vi "Signal Generator.vi"(0 "Cluster":cluster{"Frequency":dbl, "Amplitude":dbl}) -> ()   [LabVIEW 2015]
panel:
  out "error in":errorcluster
  out "error out":errorcluster
  in  "Stop":bool
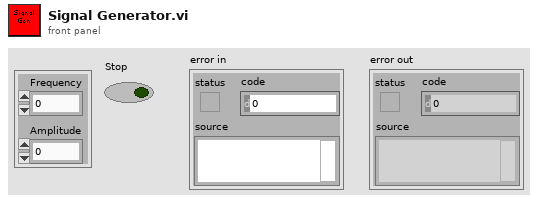
[diagram p1: front panel]
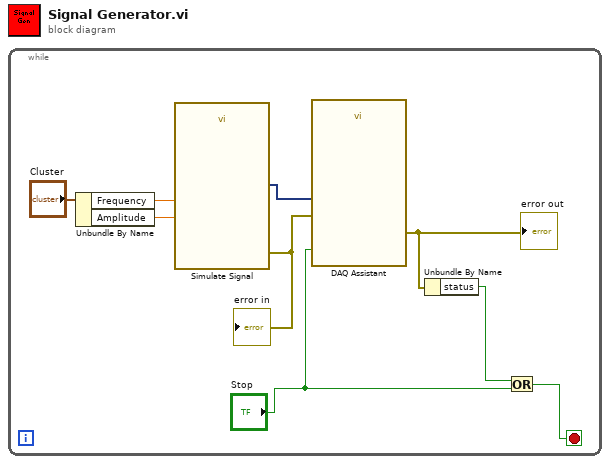
[diagram p0: block diagram]
diagram:
  n1 = while {
    stop <- w7 stop-if-true
    n2 = Unbundle By Name("Cluster") -> ("Frequency"=w2:dbl, "Amplitude"=w1:dbl)
    n3 = call "Simulate Signal"("Frequency"=w2, "Amplitude"=w1) -> ("Sine"=w4:dynamicdata, "error out"=w6:errorcluster)  [unwired: 12 in]
    "error in" <- w6
    n4 = call "DAQ Assistant"("data"=w4, "error in"=w6, "stop (F)"="Stop") -> ("error out"=w9:errorcluster)  [unwired: 14 in, 2 out]
    "error out" <- w9
    n5 = Unbundle By Name(w9) -> ("status"=w8:bool)
    n6 = Or(x=w8, y="Stop") -> (x .or. y?=w7:bool)
  }
